vi "Send_ADC.vi"(8 "error in (no error)":errorcluster, 10 "Channel":u8, 11 "Cypress in":refnum<class "Cypress.lvclass">) -> (0 "error out":errorcluster, 2 "Response":string, 3 "Cypress out":refnum<class "Cypress.lvclass">)   [LabVIEW 2019, in "Cypress.lvclass"]
uses:
  Cypress.lvclass
  Clase Padre/Serial Device.lvclass
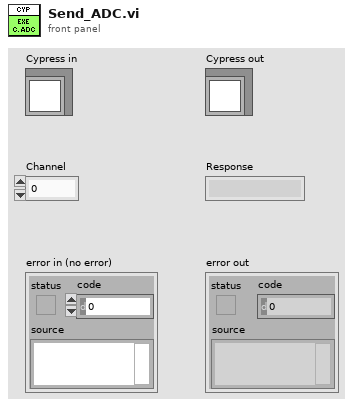
[diagram p1: front panel]
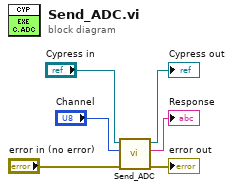
[diagram p0: block diagram]
diagram:
  n1 = call-parent "Send_ADC.vi"("error in (no error)"="error in (no error)", "Channel"="Channel", "Serial Device in"="Cypress in") -> ("error out"=→"error out":errorcluster, "Response"=→"Response":string, "Serial Device out"=→"Cypress out":refnum<class "Cypress.lvclass">)  [unwired: 6 in]
